vi "GUI_2comPort_2plot.vi"() -> ()   [LabVIEW 2018]
panel:
  in  "START / STOP":bool
  out "Particle count":dbl
  in  "?":bool
  in  "Trigger gain 2":string
  in  "Trigger level 2":string
  in  "COM-Port 2":string
  in  "?":bool
  in  "Trigger gain":string
  in  "Trigger level":string
  in  "COM-Port":string
  out "Tracer-1":dbl[](graph)
  out "Trigger":dbl[](graph)
  # "TRIGGER"
  # "TRACER-1"
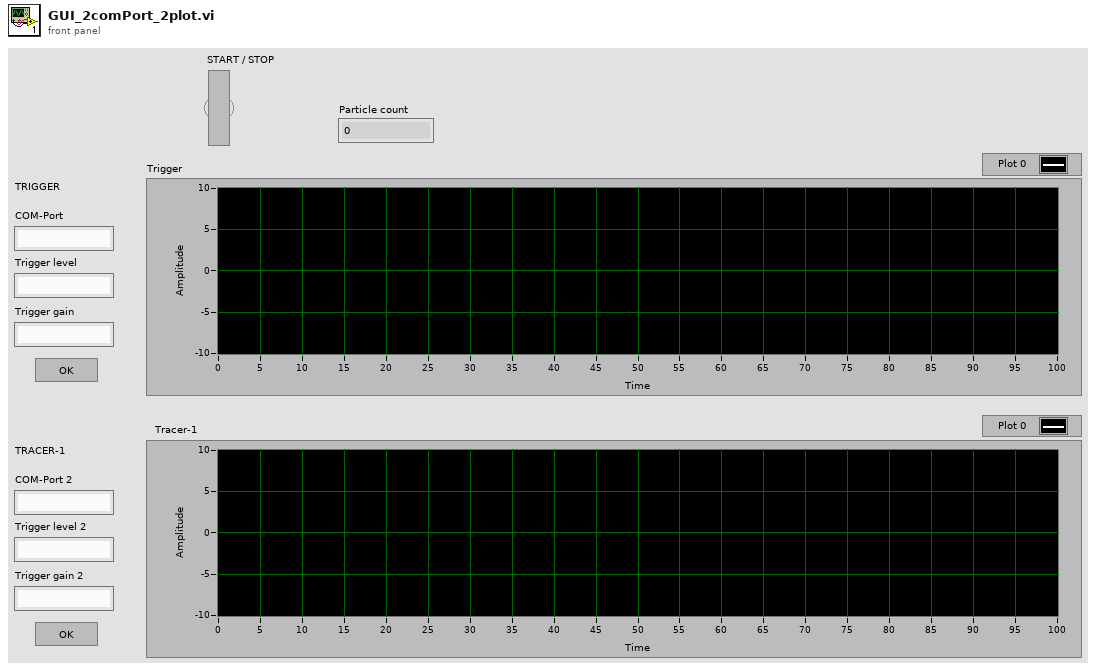
[diagram p1: front panel]
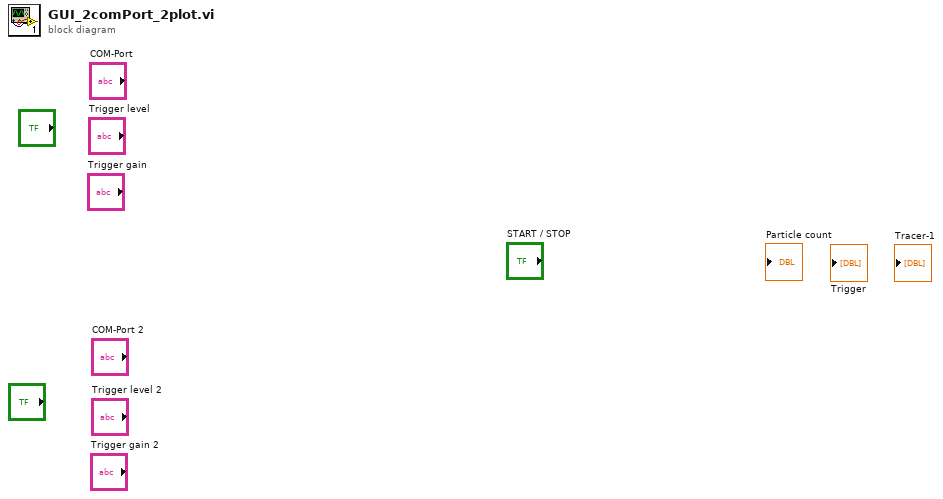
[diagram p0: block diagram]
diagram:
